vi "unescape.vi"(1 "byte array in":u8[](array[numeric]) format="%x", 2 "escape character":u8=125 format="%x") -> (0 "byte array out":u8[](array[numeric]) format="%x")   [LabVIEW 2013]
panel:
  out "Size Out":i32
  out "Size In":i32
  out "index":dbl
  # "Un-Escape\nif escape character (usually 0x7D) appears in array,\nreplace it and the next byte with that next byte xor 0x20."
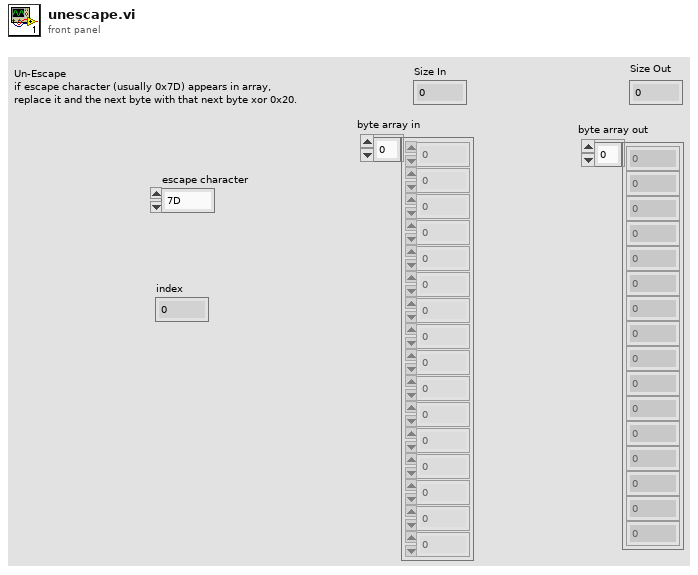
[diagram p1: front panel]
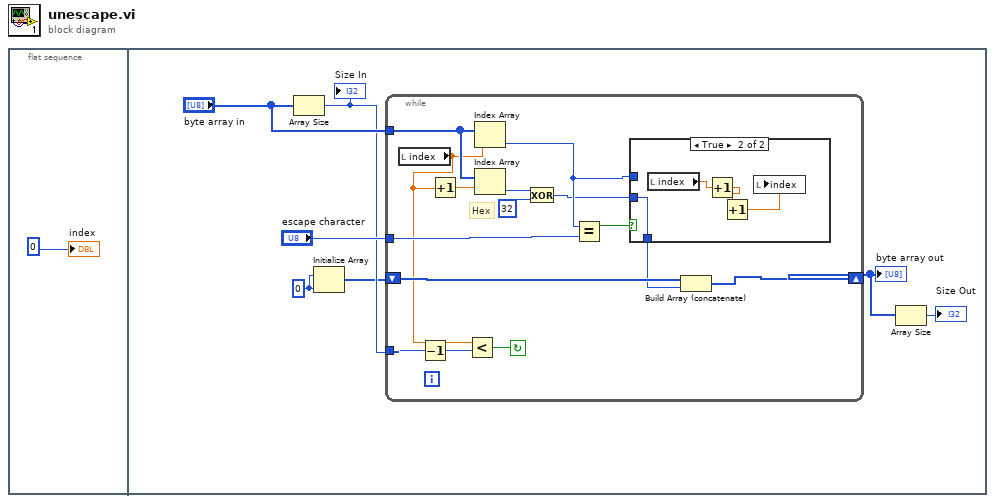
[diagram p0: block diagram]
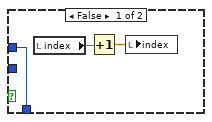
[diagram p2: hidden frame]
diagram:
  n1 = flat-sequence {
    frame #0 {
      "index" <- 0
    }
    frame #1 {
      w5 = 0 ("dimension size")
      n2 = Array Size(array="byte array in") -> (size(s)=w6:i32)
      "Size In" <- w6
      n3 = Initialize Array(w5, w5) -> (w4:i32[])
      n4 = while {
        tunnel: "escape character" -> [w23]
        tunnel: "byte array in" -> [w21]
        tunnel: w6 -> [w14]
        shift-right: [w17] -> w3
        shift-left: w4 -> [w18]
        stop <- w19 continue-if-true
        # "Hex"
        n5 = local read "index"() -> (w13:dbl)
        n6 = Decrement(x=w14) -> (x-1=w12:i32)
        n7 = Increment(x=w13) -> (x+1=w22:dbl)
        n8 = Less?(x=w13, y=w12) -> (x < y?=w19:bool)
        n9 = Index Array(array=w21, index=w13) -> (element=w16:u8)
        n10 = Index Array(array=w21, index=w22) -> (element=w9:u8)
        n11 = Exclusive Or(1:u8 32 ("y"), 2:w9) -> (0:w10:u8)
        n12 = Equal?(x=w16, y=w23) -> (x = y?=w20:bool)
        n13 = case shown="True" w20 {
          tunnel: w10 -> [_ w27]
          tunnel: w16 -> [w24 _]
          tunnel: [w24 w27] -> w15
          frame False {
            n14 = local read "index"() -> (w26:dbl)
            n15 = Increment(x=w26) -> (x+1=w25:dbl)
            n16 = local write "index"(w25) -> ()
          }
          frame True {
            n17 = local read "index"() -> (w30:dbl)
            n18 = Increment(x=w30) -> (x+1=w29:dbl)
            n19 = Increment(x=w29) -> (x+1=w28:dbl)
            n20 = local write "index"(w28) -> ()
          }
        }
        n21 = Build Array (concatenate)(w18, w15) -> (w17:i32[])
      }
      "byte array out" <- w3
      n22 = Array Size(array=w3) -> (size(s)=→"Size Out":i32)
    }
  }
